vi "Spiral Indexer.vi"(11 "Array 2":cluster{dbl, dbl}[][](array[cluster])) -> (3 "Array":cluster{dbl, dbl}[](array[cluster]))   [LabVIEW 2018]
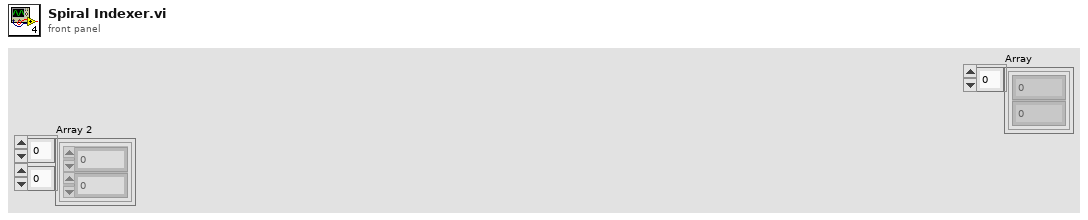
[diagram p1: front panel]
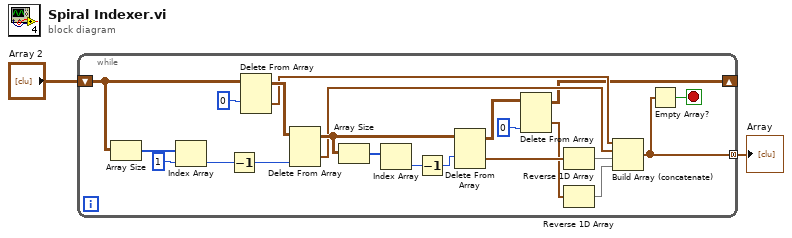
[diagram p0: block diagram]
diagram:
  n1 = while {
    shift-right: [w5] -> _
    shift-left: "Array 2" -> [w11]
    tunnel: [w13] -> w1 mode=concatenating
    stop <- w12 stop-if-true
    n2 = Array Size(array=w11) -> (size(s)=w9:i32[])
    n3 = Index Array(array=w9, index=1) -> (element=w8:i32)
    n4 = Decrement(x=w8) -> (x-1=w6:i32)
    n5 = Delete From Array(array=w11, index (row)=0) -> (deleted portion=w17:cluster{dbl, dbl}[], array with subset deleted=w24:cluster{dbl, dbl}[][])  [unwired: 2 in]
    n6 = Delete From Array(array=w24, index (col)=w6) -> (deleted portion=w16:cluster{dbl, dbl}[], array with subset deleted=w21:cluster{dbl, dbl}[][])  [unwired: 2 in]
    n7 = Array Size(array=w21) -> (size(s)=w23:i32[])
    n8 = Index Array(array=w23) -> (element=w22:i32)  [unwired: 1 in]
    n9 = Decrement(x=w22) -> (x-1=w7:i32)
    n10 = Delete From Array(array=w21, index (row)=w7) -> (deleted portion=w15:cluster{dbl, dbl}[], array with subset deleted=w20:cluster{dbl, dbl}[][])  [unwired: 2 in]
    n11 = Delete From Array(array=w20, index (col)=0 ("disabled index (col)")) -> (deleted portion=w14:cluster{dbl, dbl}[], array with subset deleted=w5:cluster{dbl, dbl}[][])  [unwired: 2 in]
    n12 = Reverse 1D Array(array=w15) -> (reversed array=w4:cluster{dbl, dbl}[])
    n13 = Reverse 1D Array(array=w14) -> (reversed array=w3:cluster{dbl, dbl}[])
    n14 = Build Array (concatenate)(w17, w16, w4, w3) -> (w13:cluster{dbl, dbl}[])
    n15 = Empty Array?(array=w13) -> (empty?=w12:bool)
  }
  "Array" <- w1
